vi "Robot_Simulation_Listen_Connect.vi"(8 "error in (no error)":errorcluster, 10 "timeout ms (25000)":i32=25000, 11 "port":u16=3300) -> (0 "error out":errorcluster, 1 "Properties:Request URI":string, 2 "Properties:Return Headers":variant, 3 "WebSocket Connection out":refnum<class "WebSocket Server.lvclass">)   [LabVIEW 2019]
uses:
  <vilib>/MediaMongrels Ltd/WebSockets/WebSockets/WebSocket Server/WebSocket Server.lvclass
  C:/Program Files/National Instruments/LabVIEW 2019/vi.lib/MediaMongrels Ltd/WebSockets/WebSockets/WebSocket/WebSocket.lvclass
  <vilib>/MediaMongrels Ltd/WebSockets/WebSockets/WebSocket/WebSocket.lvclass/WebSocket.ctl
  <vilib>/MediaMongrels Ltd/WebSockets/WebSockets/WebSocket Server/WebSocket Server.lvclass/WebSocket Server.ctl
  <vilib>/MediaMongrels Ltd/WebSockets/WebSockets/WebSocket/Read Return Headers.vi
  <vilib>/MediaMongrels Ltd/WebSockets/WebSockets/WebSocket Server/Read Request URI.vi
  <vilib>/MediaMongrels Ltd/WebSockets/Sockets/VISA TCP Socket/VISA TCP.lvclass
  C:/Program Files/National Instruments/LabVIEW 2019/vi.lib/MediaMongrels Ltd/WebSockets/Sockets/Socket/Socket.lvclass
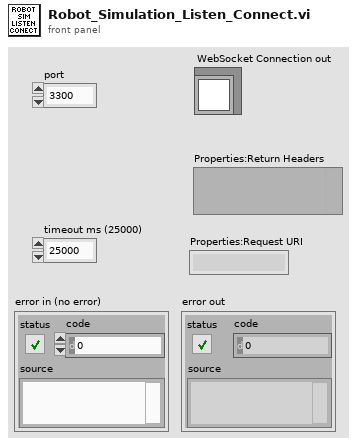
[diagram p1: front panel]
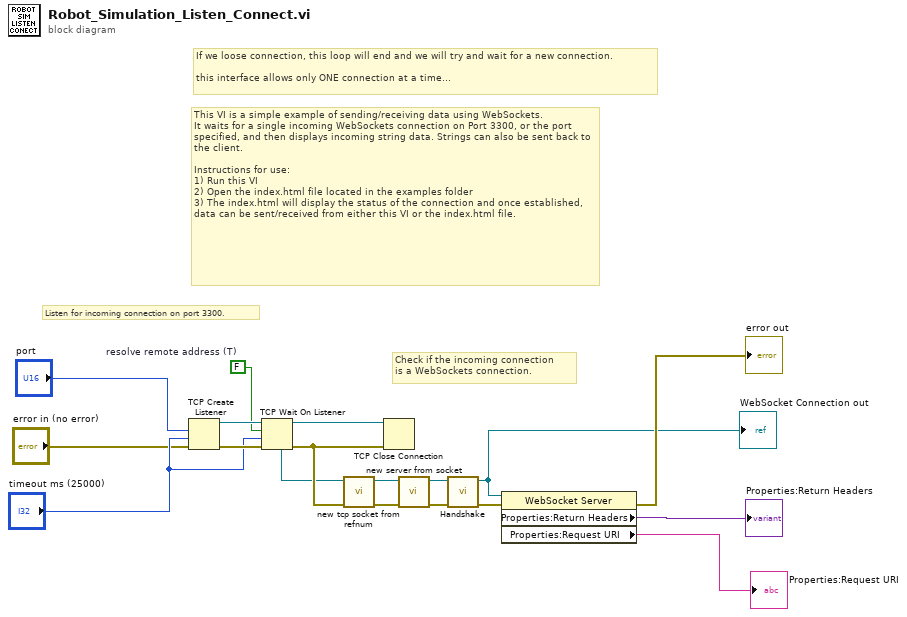
[diagram p0: block diagram]
diagram:
  w2 = FALSE  # resolve remote address (T)
  # "If we loose connection, this loop will end and we will try and wait for a new connection.\n\nthis interface allows only ONE connection at a time..."
  # "This VI is a simple example of sending/receiving data using WebSockets.\nIt waits for a single incoming WebSockets connection on Port 3300, or the port specified, and then displays incoming string data. Strings can also be sent back to the client.\n\nInstructions for use:\n1) Run this VI\n2) Open the index.html file located in the examples folder\n3) The index.html will display the status of the connection and once established, data can be sent/received from either this VI or the index.html file."
  # "Check if the incoming connection\nis a WebSockets connection."
  # "Listen for incoming connection on port 3300."
  n1 = TCP Create Listener(8:"error in (no error)", 9:"timeout ms (25000)", 10:"port") -> (0:w11:errorcluster, 3:w10:refnum<k5>)  [unwired: 2 in, 1 out]
  n2 = TCP Wait On Listener(8:w11, 9:"timeout ms (25000)", 10:w2, 11:w10) -> (0:w8:errorcluster, 3:w6:refnum<k5>, 4:w3:refnum<k5>)  [unwired: 2 out]
  n3 = call <vilib>:"new tcp socket from refnum.vi"("error in (no error)"=w8, "TCP Network Connection Refnum"=w3) -> ("error out"=w4:errorcluster, "VISA TCP out"=w5:refnum<class "VISA TCP.lvclass">)  [unwired: 8 in]
  n4 = TCP Close Connection(connection ID=w6, error in (no error)=w8) -> ()  [unwired: 1 in, 2 out]
  n5 = call <vilib>:"new server from socket.vi"("error in (no error)"=w4, "Socket"=w5) -> ("error out"=w16:errorcluster, "WebSocket Server out"=w15:refnum<class "WebSocket Server.lvclass">)  [unwired: 8 in]
  n6 = call-dynamic "Handshake.vi"("error in (no error)"=w16, "WebSocket Connection in"=w15) -> ("error out"=w14:errorcluster, "WebSocket Connection out"=w1:refnum<class "WebSocket Server.lvclass">)  [unwired: 8 in]
  "WebSocket Connection out" <- w1
  n7 = property class="WebSocket Server"(reference=w1, error in=w14) -> (error out=→"error out":errorcluster, "Properties:Return Headers"=→"Properties:Return Headers":variant, "Properties:Request URI"=→"Properties:Request URI":string)  [unwired: 1 out]
